vi "generic_array_average.vi"(1 "Array int 32":i32[][](array[numeric])) -> (0 "Average":ext format="%.2f")   [LabVIEW 2013]
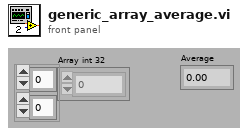
[diagram p1: front panel]
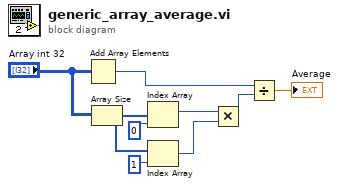
[diagram p0: block diagram]
diagram:
  n1 = Add Array Elements(numeric array="Array int 32") -> (sum=w1:i32)
  n2 = Array Size(array="Array int 32") -> (size(s)=w5:i32[])
  n3 = Index Array(array=w5, index=0) -> (element=w8:i32)
  n4 = Index Array(array=w5, index=1) -> (element=w9:i32)
  n5 = Multiply(x=w8, y=w9) -> (x*y=w3:i32)
  n6 = Divide(x=w1, y=w3) -> (x/y=→"Average":dbl)
